vi "MyMPHTask.vi"(8 "error in":errorcluster) -> (0 "error out":errorcluster, 3 "task out":refnum<k21>)   [LabVIEW 2020]
uses:
  <vilib>/DAQmx/create/channels.llb/DAQmx Create Channel (CI-Velocity-Linear).vi
  <vilib>/DAQmx/configure/timing.llb/DAQmx Timing (Sample Clock).vi
  <resource>/objmgr/daqmx.rc
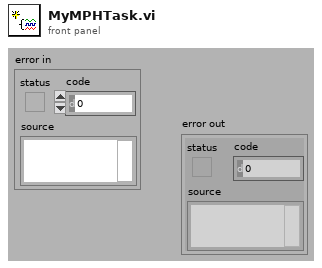
[diagram p1: front panel]
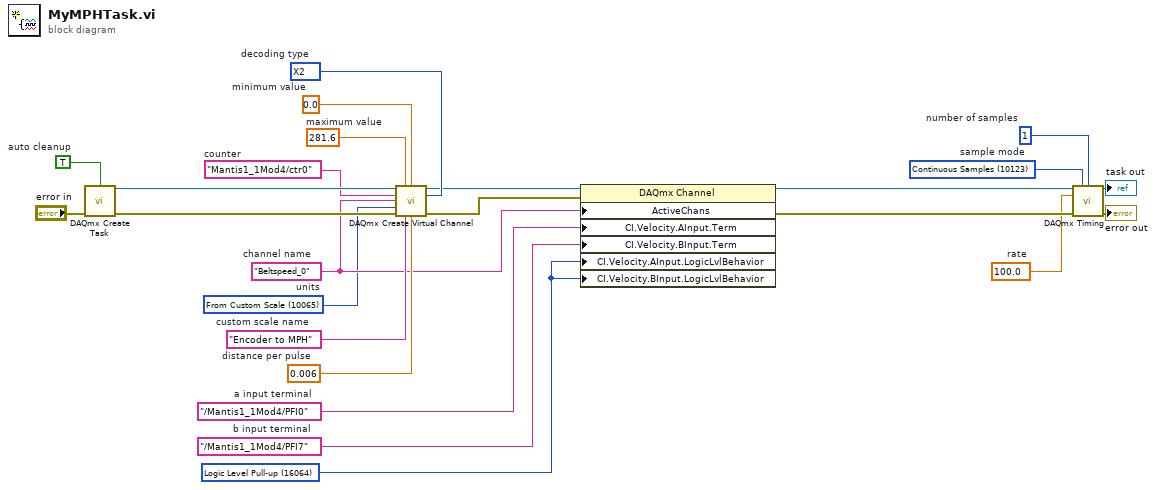
[diagram p0: block diagram]
diagram:
  w1 = 16064 items=["Logic Level Pull-up"=16064, "None"=10230] ("CI.Velocity.AInput.LogicLvlBehavior")
  w2 = 10123 items=["Finite Samples"=10178, "Continuous Samples"=10123, "Hardware Timed Single Point"=12522]  # sample mode
  w3 = 1  # number of samples
  w4 = 100.0  # rate
  w9 = 10065 items=["in/s"=15960, "m/s"=15959, "From Custom Scale"=10065]  # units
  w12 = "/Mantis1_1Mod4/PFI7"  # b input terminal
  w13 = "/Mantis1_1Mod4/PFI0"  # a input terminal
  w15 = 10091 items=["X1"=10090, "X2"=10091, "X4"=10092, "Two Pulse Counting"=10313]  # decoding type
  w16 = 0.006  # distance per pulse
  w17 = "Encoder to MPH"  # custom scale name
  w18 = 0.0  # minimum value
  w8 = 281.6  # maximum value
  w11 = "Beltspeed_0"  # channel name
  w20 = "Mantis1_1Mod4/ctr0"  # counter
  w22 = TRUE  # auto cleanup
  n1 = call <vilib>:"DAQmx Create Task.vi"("auto cleanup"=w22, "error in"="error in") -> ("task out"=w21:refnum<k21>, "error out"=w23:errorcluster)  [unwired: 12 in]
  n2 = call-poly <vilib>:"DAQmx Create Virtual Channel.vi"("task in"=w21, "maximum value"=w8, "minimum value"=w18, "counter"=w20, "decoding type"=w15, "name to assign"=w11, "units"=w9, "error in"=w23, "custom scale name"=w17, "distance per pulse"=w16) -> ("task out"=w14:refnum<k21>, "error out"=w19:errorcluster)  [unwired: 4 in]
  n3 = property class="DAQmx Channel"(reference=w14, error in=w19, "ActiveChans"=w11, "CI.Velocity.AInput.Term"=w13, "CI.Velocity.BInput.Term"=w12, "CI.Velocity.AInput.LogicLvlBehavior"=w1, "CI.Velocity.BInput.LogicLvlBehavior"=w1) -> (reference out=w5:refnum<k21>, error out=w10:errorcluster)
  n4 = call-poly <vilib>:"DAQmx Timing.vi"("task/channels in"=w5, "sample mode"=w2, "samples per channel"=w3, "rate"=w4, "error in"=w10) -> ("task out"=→"task out":refnum<k21>, "error out"=→"error out":errorcluster)  [unwired: 9 in]
